vi "Fetch Array.vi"(8 "error in (no error)":errorcluster {"code" format="%.0x"}, 9 "Measurement Type  (1: Voltage)":i32(ring)=1 items=["Current", "Voltage", "Power"], 10 "Channel Name (1)":string="1", 11 "VISA resource name":refnum<visa-resource-name>) -> (0 "error out":errorcluster {"code" format="%.0x"}, 1 "Actual Points":i32, 2 "Measurement Array":dbl[](array[numeric]) format="%^.3e", 3 "VISA resource name out":refnum<visa-resource-name>)   [LabVIEW 2018, in "Agilent N6700 Series.lvlib"]
doc: "Returns the measurement the DC Power supply acquires for the channel you specify. The waveform is from an acquisition that you previously initiated. \n\n<b>Note:</b>\nThis VI only applies to models N676xA, N678xA SMU, or models N673xA. N674xA, N675xA, and N677xA with Option 054 (High Speed Test Extensions)."
uses:
  Agilent N6700 Series.lvlib
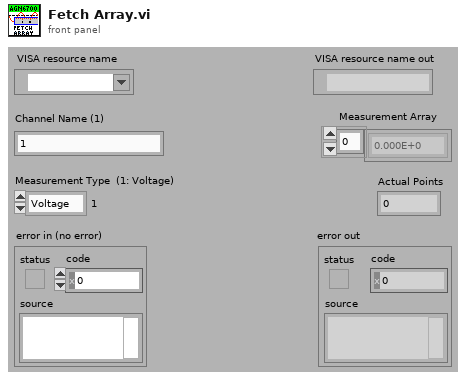
[diagram p1: front panel]
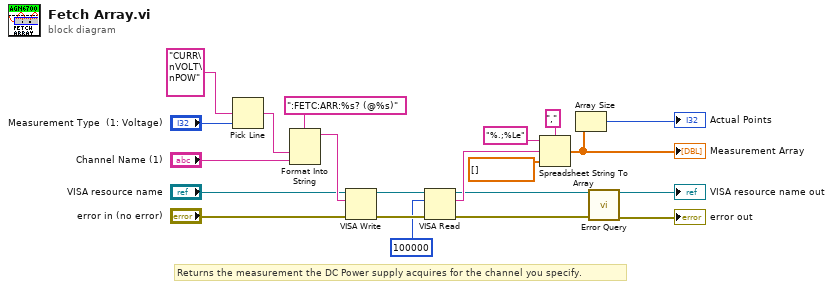
[diagram p0: block diagram]
diagram:
  # "Returns the measurement the DC Power supply acquires for the channel you specify."
  n1 = Pick Line(multi-line string="CURR\nVOLT\nPOW", line index="Measurement Type  (1: Voltage)") -> (output string=w16:string)  [unwired: 1 in]
  n2 = Format Into String(format string=":FETC:ARR:%s? (@%s)", w16, "Channel Name (1)") -> (resulting string=w18:string)  [unwired: 2 in, 1 out]
  n3 = VISA Write(VISA resource name="VISA resource name", write buffer=w18, error in (no error)="error in (no error)") -> (VISA resource name out=w21:refnum<visa-resource-name>, error out=w20:errorcluster)  [unwired: 1 out]
  n4 = VISA Read(VISA resource name=w21, byte count=100000 ("Array Size"), error in (no error)=w20) -> (VISA resource name out=w2:refnum<visa-resource-name>, read buffer=w12:string, error out=w1:errorcluster)  [unwired: 1 out]
  n5 = Spreadsheet String To Array(delimiter (Tab)=",", format string="%.;%Le", spreadsheet string=w12, array type (2D Dbl)=dbl[] []) -> (array=w11:dbl[])
  "Measurement Array" <- w11
  n6 = Array Size(array=w11) -> (size(s)=→"Actual Points":i32)
  n7 = call "Error Query.vi"("VISA resource name"=w2, "error in (no error)"=w1) -> ("VISA resource name out"=→"VISA resource name out":refnum<visa-resource-name>, "error out"=→"error out":errorcluster)  [unwired: 10 in, 2 out]
